vi "Proy2.1.vi"() -> ()   [LabVIEW 2022 SP3]
uses:
  <vilib>/addons/_XControls/Function Generator Configuration/Test Signal Configuration.xctl
  <vilib>/addons/_NISVFA/_Generation/Signal Generation/SV Signal/SV Signal.lvclass
  <vilib>/addons/_NISVFA/_Generation/Signal Generation/SV Signal/sv_System Timing Model.ctl
  5e9e65be-7a47-452a-902e-fe4f03c459fa.vi
  <vilib>/DAQmx/write.llb/DAQmx Write (Analog Wfm 1Chan NSamp).vi
  <vilib>/DAQmx/create/channels.llb/DAQmx Create Channel (AO-Voltage-Basic).vi
  <vilib>/DAQmx/configure/timing.llb/DAQmx Timing (Sample Clock).vi
  <vilib>/addons/_NISVFA/_Generation/Signal Generation/SV Signal/Write Sample Rate.vi
  <vilib>/addons/_NISVFA/_Generation/Signal Generation/SV Signal/Write System Timing Model.vi
  <vilib>/addons/_NISVFA/_Generation/Signal Generation/SV Signal/Write Ramp Parameters.vi
  <vilib>/addons/_NISVFA/_Generation/Signal Generation/SV Signal/Write Maximum Value.vi
  <vilib>/addons/_NISVFA/_Generation/Signal Generation/SV Signal/Write Minimum Value.vi
  <vilib>/DAQmx/miscellaneous.llb/DAQmx Fill In Error Info.vi
  <resource>/objmgr/daqmx.rc
panel:
  out "Filename Out 2":path caption="Filename Out"
  in  "myDAQ Max, AO":dbl(slide) scale=0.0..10.0
  in  "signal configuration":refnum<class "SV Signal.lvclass">(xcontrol)
  in  "physical channels":tag="Dev1/ao0"
  out "Waveform":waveform(dbl)(graph)
  in  "stop":bool
  out "error out":errorcluster
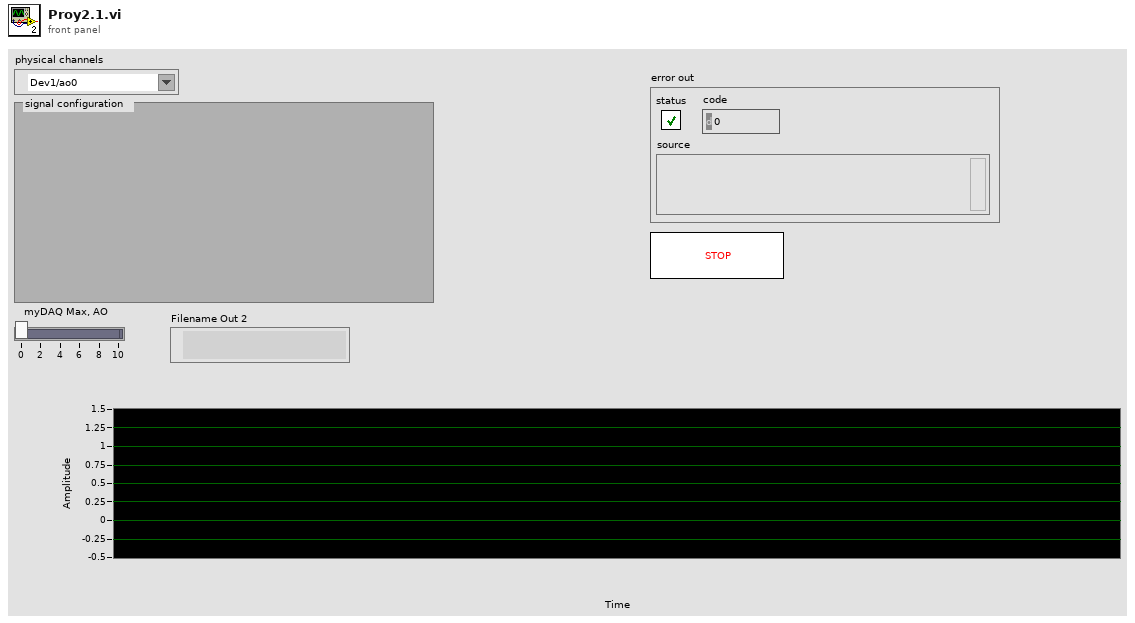
[diagram p1: front panel]
types:
  T1 = cluster{"profile":enum16{"Linear", "Half cosine"}, "durations [s]":cluster{"ramp-up":dbl, "transition":dbl, "ramp-down":dbl}}
  T2 = typedef "SV Signal.lvclass/sv_System Timing Model.ctl" = i64
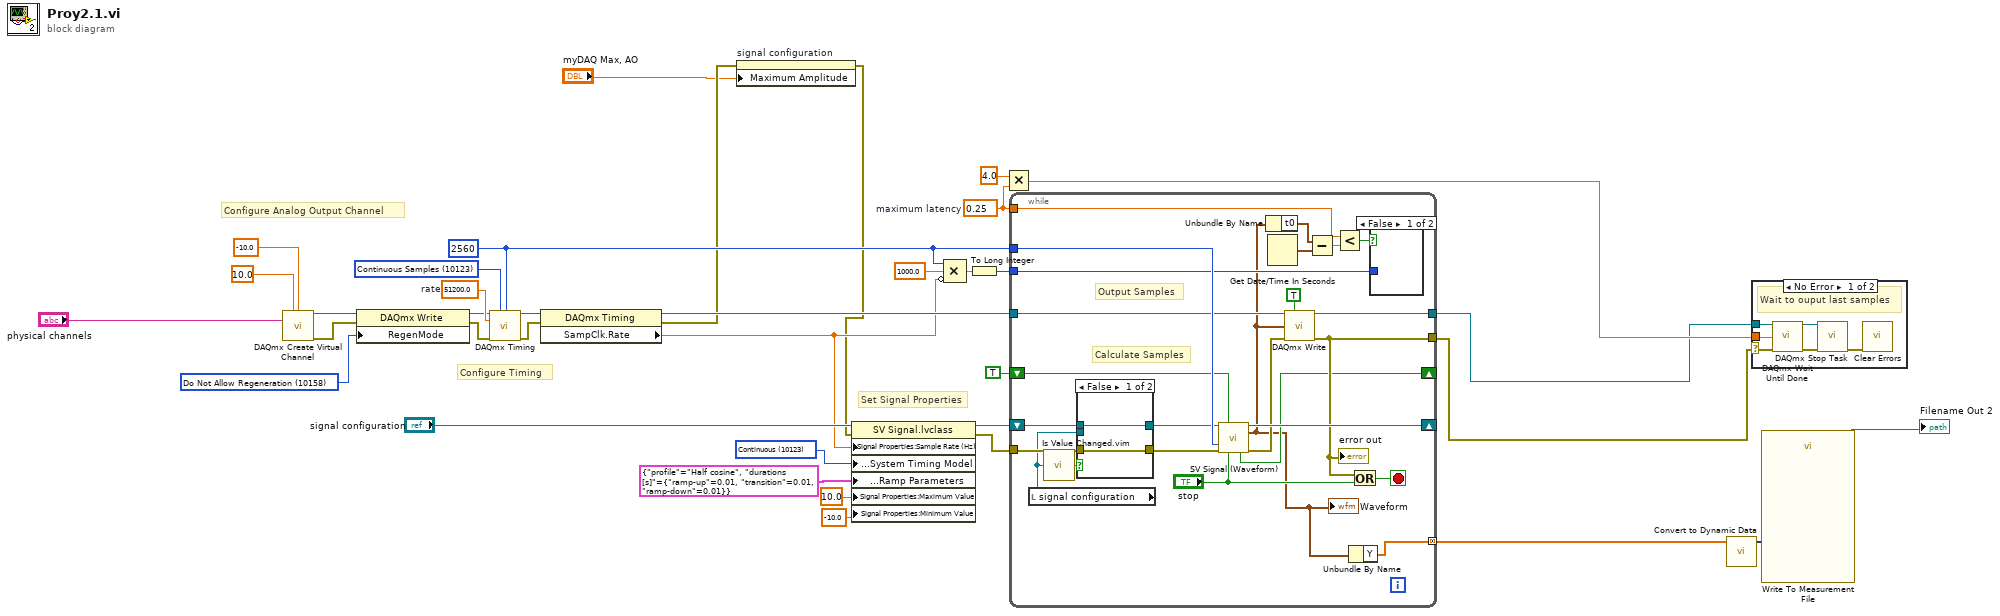
[diagram p0: block diagram]
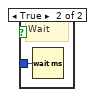
[diagram p3: hidden frame]
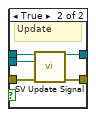
[diagram p4: hidden frame]
diagram:
  w14 = 0.25  # maximum latency
  w27 = 10158 items=["Allow Regeneration"=10097, "Do Not Allow Regeneration"=10158] ("RegenMode")
  w16 = 2560 ("samples per channel")
  w31 = 10123 items=["Finite Samples"=10178, "Continuous Samples"=10123, "Hardware Timed Single Point"=12522] ("sample mode")
  w32 = 51200.0  # rate
  w35 = T2 10123 items=["Finite"=10178, "-"=-1, "Continuous"=10123, "-"=-2, "Settled"=110123, "Averaged"=210123, "Discrete Sweep"=310123, "Continuous Sweep"=410123] ("System Timing Model")
  # "Configure Timing"
  # "Configure Analog Output Channel"
  # "Set Signal Properties"
  n1 = call-poly <vilib>:"DAQmx Create Virtual Channel.vi"("maximum value"=10.0, "minimum value"=-10.0, "physical channels"="physical channels") -> ("task out"=w26:refnum<k21>, "error out"=w24:errorcluster)  [unwired: 11 in]
  n2 = property class="DAQmx Write"(reference=w26, error in=w24, "RegenMode"=w27) -> (reference out=w25:refnum<k21>, error out=w23:errorcluster)
  n3 = call-poly <vilib>:"DAQmx Timing.vi"("task/channels in"=w25, "sample mode"=w31, "samples per channel"=w16, "rate"=w32, "error in"=w23) -> ("task out"=w33:refnum<k21>, "error out"=w29:errorcluster)  [unwired: 9 in]
  n4 = property class="DAQmx Timing"(reference=w33, error in=w29) -> (reference out=w30:refnum<k21>, error out=w12:errorcluster, "SampClk.Rate"=w17:dbl)
  n5 = property on="signal configuration" class="Test Signal Configuration (stri"(error in=w12, "Maximum Amplitude"="myDAQ Max, AO") -> (error out=w11:errorcluster)  [unwired: 1 in, 1 out]
  n6 = property class="SV Signal.lvclass"(reference="signal configuration", error in=w11, "Signal Properties:Sample Rate (Hz)"=w17, "Signal Properties:System Timing Model"=w35, "Signal Properties:Ramps:Ramp Parameters"=T1 {"profile"=enum."Half cosine", "durations [s]"={"ramp-up"=0.01, "transition"=0.01, "ramp-down"=0.01}} ("Ramp Parameters:All Elements"), "Signal Properties:Maximum Value"=10.0 ("Maximum Value"), "Signal Properties:Minimum Value"=-10.0 ("Minimum Value")) -> (reference out=w36:refnum<class "SV Signal.lvclass">, error out=w37:errorcluster)
  n7 = Compound Arithmetic op=MULTIPLY(w16, 1000.0 ("value"), invert w17) -> (w19:dbl)
  n8 = To Long Integer(number=w19) -> (32bit integer=w13:i32)
  n9 = Multiply(x=4.0 ("value"), y=w14) -> (x*y=w4:dbl)
  n10 = while {
    tunnel: w37 -> [w53]
    shift-right: [w62] -> _
    shift-left: w36 -> [w54]
    tunnel: w16 -> [w60]
    tunnel: w30 -> [w59]
    tunnel: [w40] -> w3
    tunnel: [w56] -> w5
    shift-right: [w47] -> _
    shift-left: TRUE ("done") -> [w49]
    tunnel: w14 -> [w42]
    tunnel: w13 -> [w41]
    tunnel: [w38] -> w2 mode=concatenating
    stop <- w61 stop-if-true
    # "Output Samples"
    # "Calculate Samples"
    n11 = local read "signal configuration"() -> (w50:refnum<class "SV Signal.lvclass">)
    n12 = call "Is Value Changed.vim"("value"=w50) -> ("changed or first call?"=w55:bool)
    n13 = case shown="False" w55 {
      tunnel: w54 -> [w65 w70]
      tunnel: w53 -> [w64 w69]
      tunnel: [w64 w68] -> w52
      tunnel: [w65 w67] -> w51
      tunnel: w50 -> [_ w66]
      frame False {
      }
      frame True {
        # "Update"
        n14 = call-dynamic "SV Update Signal.vi"("current configuration"=w70, "new configuration"=w66, "error in (no error)"=w69) -> ("updated configuration"=w67:refnum<class "SV Signal.lvclass">, "error out"=w68:errorcluster)  [unwired: 11 in]
      }
    }
    n15 = call-dynamic "SV Signal (Waveform).vi"("signal configuration"=w51, "reset"=w49, "samples"=w60, "error in (no error)"=w52, "stop"="stop") -> ("signal configuration"=w62:refnum<class "SV Signal.lvclass">, "output waveform"=w39:waveform(dbl), "done"=w47:bool, "error out"=w58:errorcluster)  [unwired: 5 in, 2 out]
    "Waveform" <- w39
    n16 = Unbundle By Name(w39) -> ("t0"=w46:timestamp)
    n17 = Get Date/Time In Seconds() -> (seconds since 1Jan1904=w45:timestamp)
    n18 = call-poly <vilib>:"DAQmx Write.vi"("task/channels in"=w59, "auto start"=TRUE, "data"=w39, "error in"=w58) -> ("task out"=w40:refnum<k21>, "error out"=w56:errorcluster)  [unwired: 9 in, 1 out]
    "error out" <- w56
    n19 = Subtract(x=w46, y=w45) -> (x-y=w44:dbl)
    n20 = Less?(x=w42, y=w44) -> (x < y?=w43:bool)
    n21 = Unbundle By Name(w39) -> ("Y"=w38:dbl[])
    n22 = Or(x=w56, y="stop") -> (x .or. y?=w61:bool)
    n23 = case shown="False" w43 {
      tunnel: w41 -> [_ w63]
      frame False {
      }
      frame True {
        # "Wait"
        n24 = Wait (ms)(milliseconds to wait=w63) -> ()  [unwired: 1 out]
      }
    }
  }
  n25 = call "Convert to Dynamic Data"("Array"=w2) -> ("Dynamic Data Type"=w1:dynamicdata)  [unwired: 3 in]
  n26 = case shown="No Error" w5 {
    selector: w5 -> [w73 _]
    tunnel: w3 -> [w76 _]
    tunnel: w4 -> [w71 _]
    frame No Error {
      # "Wait to ouput last samples"
      n27 = call <vilib>:"DAQmx Wait Until Done.vi"("task/channels in"=w76, "timeout (sec)"=w71, "error in"=w73) -> ("task out"=w75:refnum<k21>, "error out"=w74:errorcluster)  [unwired: 11 in]
      n28 = call <vilib>:"DAQmx Stop Task.vi"("task/channels in"=w75, "error in"=w74) -> ("error out"=w72:errorcluster)  [unwired: 12 in, 1 out]
      n29 = call <vilib>:"Clear Errors.vi"("error in (no error)"=w72) -> ()  [unwired: 5 in, 2 out]
    }
    frame Error {
    }
  }
  n30 = call "Write To Measurement File"("Signals"=w1) -> ("Filename Out"=→"Filename Out 2":path)  [unwired: 16 in, 2 out]
